vi "Read Filename.vi"(8 "error in (no error)":errorcluster, 11 "Process Settings in":refnum<class "Process Settings.lvclass">) -> (0 "error out":errorcluster, 2 "Filename":path, 3 "Process Settings out":refnum<class "Process Settings.lvclass">)   [LabVIEW 2017, in "Process Settings.lvclass"]
uses:
  Process Settings.lvclass
  Process Settings.lvclass/Process Settings.ctl
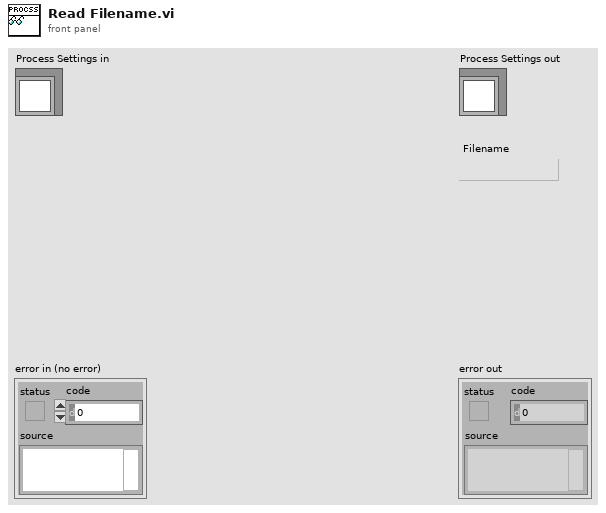
[diagram p1: front panel]
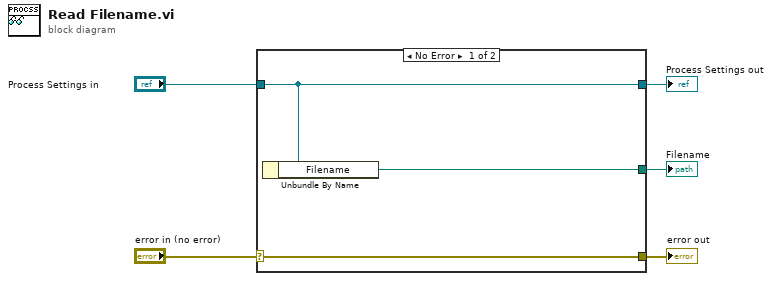
[diagram p0: block diagram]
diagram:
  n1 = case shown="No Error" "error in (no error)" {
    selector: "error in (no error)" -> [w8 w9]
    tunnel: [w8 w9] -> w4
    tunnel: [w7 w10] -> w2
    tunnel: "Process Settings in" -> [w7 w10]
    tunnel: [w6 _] -> w1
    frame No Error {
      n2 = Unbundle By Name(w7) -> ("Filename"=w6:path)
    }
    frame Error {
    }
  }
  "error out" <- w4
  "Process Settings out" <- w2
  "Filename" <- w1
